vi "Dirac Integrand for Gated Decay.vi"(8 "Error In":errorcluster, 11 "data":variant) -> (0 "Error Out":errorcluster, 3 "F(X)":dbl)   [LabVIEW 2019]
doc: "This template is the starting point for creating a function that is the integrand evaluation to be passed to the Quadrature.vi."
uses:
  Gate & Decay Parameters.ctl
  Gate Type.ctl
  IRF Model.ctl
  XY Plot Data.ctl
  <vilib>/Utility/error.llb/Error Cluster From Error Code.vi
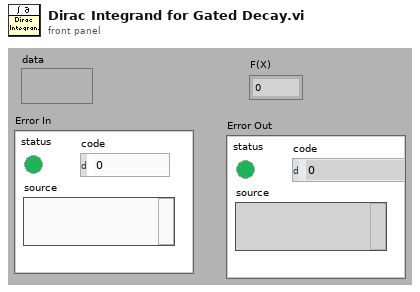
[diagram p1: front panel]
types:
  T1 = typedef "Gate & Decay Parameters.ctl" = cluster{"W":dbl, "T":dbl, "tau":dbl, "t_0":dbl, "Gate Type":T2, "t_i":dbl, "sR":dbl, "sF":dbl, "s":dbl, "Reversed Sawtooth":bool, "IRF Model":T3, "IRF Parameter 1":dbl, "User-defined Gate":T4, "Type of User-defined Function":enum32{"Gate", "IRF"}}
  T2 = typedef "Gate Type.ctl" = enum16{"Square", "Finite Edge Square", "Finite Edge, Tilted Top Square", "Triangle", "Sawtooth", "User-defined"}
  T3 = typedef "IRF Model.ctl" = enum16{"Dirac", "Exponential"}
  T4 = typedef "XY Plot Data.ctl" = cluster{"X Array":dbl[], "Y Array":dbl[]}
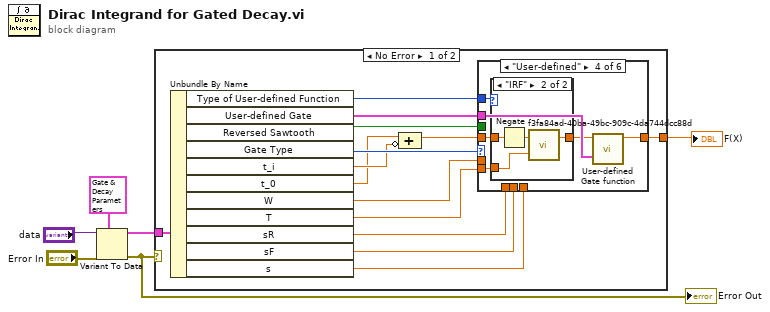
[diagram p0: block diagram]
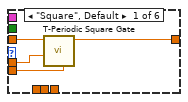
[diagram p2: hidden frame]
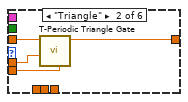
[diagram p3: hidden frame]
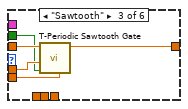
[diagram p4: hidden frame]
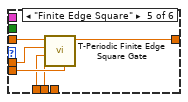
[diagram p6: hidden frame]
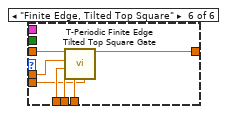
[diagram p7: hidden frame]
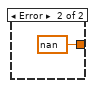
[diagram p8: hidden frame]
diagram:
  n1 = Variant To Data(error in="Error In", type=T1 {"W"=0.0, "T"=0.0, "tau"=0.0, "t_0"=0.0, "Gate Type"=enum."Square", "t_i"=0.0, "sR"=0.0, "sF"=0.0, "s"=0.0, "Reversed Sawtooth"=FALSE, "IRF Model"=enum."Dirac", "IRF Parameter 1"=0.0, "User-defined Gate"={"X Array"=[], "Y Array"=[]}, "Type of User-defined Function"=enum."Gate"} ("Gate & Decay Parameters"), Variant="data") -> (data=w4:T1, error out=w1:errorcluster)
  "Error Out" <- w1
  n2 = case shown="No Error" w1 {
    tunnel: w4 -> [w10 _]
    tunnel: [w7 nan ("Finite Edge Square(t)")] -> w3
    frame No Error {
      n3 = Unbundle By Name(w10) -> ("Type of User-defined Function"=w9:enum32{"Gate", "IRF"}, "User-defined Gate"=w11:T4, "Reversed Sawtooth"=w12:bool, "Gate Type"=w19:T2, "t_i"=w18:dbl, "t_0"=w8:dbl, "W"=w16:dbl, "T"=w20:dbl, "sR"=w15:dbl, "sF"=w14:dbl, "s"=w13:dbl)
      n4 = Compound Arithmetic op=ADD(w8, invert w18) -> (w17:dbl)
      n5 = case shown="\"User-defined\"" w19 {
        tunnel: w16 -> [w23 w28 w32 _ w48 w55]
        tunnel: w17 -> [w24 w27 w33 w39 w50 w57]
        tunnel: [w22 w26 w31 w38 w49 w56] -> w7
        tunnel: w15 -> [_ _ _ _ w46 w54]
        tunnel: w14 -> [_ _ _ _ w45 w53]
        tunnel: w13 -> [_ _ _ _ _ w52]
        tunnel: w12 -> [_ _ w30 _ _ _]
        tunnel: w11 -> [_ _ _ w37 _ _]
        tunnel: w20 -> [w21 w25 w29 w36 w47 w51]
        tunnel: w9 -> [_ _ _ w34 _ _]
        frame "Square", Default {
          n6 = call "T-Periodic Square Gate.vi"("Period T"=w21, "W"=w23, "t"=w24) -> ("Square(t)"=w22:dbl)  [unwired: 8 in]
        }
        frame "Triangle" {
          n7 = call "T-Periodic Triangle Gate.vi"("Period T"=w25, "W"=w28, "t"=w27) -> ("Triangle(t)"=w26:dbl)  [unwired: 8 in]
        }
        frame "Sawtooth" {
          n8 = call "T-Periodic Sawtooth Gate.vi"("Period T"=w29, "Reversed?"=w30, "W"=w32, "t"=w33) -> ("Sawtooth(t)"=w31:dbl)  [unwired: 7 in]
        }
        frame "User-defined" {
          n9 = case shown="\"IRF\"" w34 {
            tunnel: w39 -> [w40 w44]
            tunnel: w36 -> [_ w42]
            tunnel: [w40 w41] -> w35
            frame "Gate", Default {
            }
            frame "IRF" {
              n10 = Negate(x=w44) -> (-x=w43:dbl)
              n11 = call "f3fa84ad-40ba-49bc-909c-4da744dcc88d.vi"("y"=w42, "x"=w43) -> ("x - E(x/y)y"=w41:dbl)  [unwired: 1 out]
            }
          }
          n12 = call "User-defined Gate function.vi"("User-defined Gate"=w37, "t"=w35) -> ("User-defined Gate(t)"=w38:dbl)  [unwired: 8 in, 1 out]
        }
        frame "Finite Edge Square" {
          n13 = call "T-Periodic Finite Edge Square Gate.vi"("Period T"=w47, "s_F"=w45, "s_R"=w46, "W"=w48, "t"=w50) -> ("Finite Edge Square(t)"=w49:dbl)  [unwired: 6 in]
        }
        frame "Finite Edge, Tilted Top Square" {
          n14 = call "T-Periodic Finite Edge Tilted Top Square Gate.vi"("Period T"=w51, "slope"=w52, "s_F"=w53, "s_R"=w54, "W"=w55, "t"=w57) -> ("Finite Edge Square(t)"=w56:dbl)  [unwired: 5 in]
        }
      }
    }
    frame Error {
    }
  }
  "F(X)" <- w3
